vi "ReadGroup.vi"(7 "LabVIEW Web Service Request":refnum<class "Web Request.lvclass">, 11 "groupName":string) -> ()   [LabVIEW 2013]
doc: "Read group returns the values of all the tags in a specified group."
uses:
  <vilib>/wsapi/Web Request.lvclass
  <vilib>/NI/TagWebClient/API/JSON Formats/ReadGroup Results.ctl
  <vilib>/NI/TagWebClient/API/JSON Formats/group type.ctl
  <vilib>/NI/TagWebClient/API/tagweb client API.lvlib
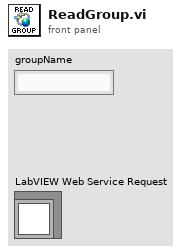
[diagram p1: front panel]
types:
  T1 = typedef "tagweb client API.lvlib/ReadGroup Results.ctl" = cluster{"data":T2[]}
  T2 = typedef "tagweb client API.lvlib/group type.ctl" = cluster{"type":string, "Values":string[]}
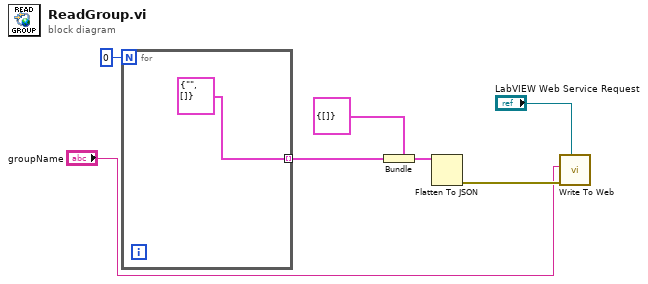
[diagram p0: block diagram]
diagram:
  n1 = for {
    N: 0 -> [_]
    tunnel: [T2 {"type"="", "Values"=[]} ("Cluster")] -> w3 mode=indexing
  }
  n2 = Bundle(cluster=T1 {"data"=[]} ("Read Group Results"), "data"=w3) -> (w6:T1)
  n3 = Flatten To JSON(anything=w6) -> (11:w7:errorcluster)  [unwired: 2 in, 1 out]
  n4 = call <vilib>:"Write To Web.vi"("Web Request in"="LabVIEW Web Service Request", "error in"=w7, "Response String"="groupName") -> ()  [unwired: 9 in]
